vi "Bind SQL Parameters.vi"   [LabVIEW 2023, in "SQLite DB Operator.lvclass"]
uses:
  SQLite DB Operator.lvclass
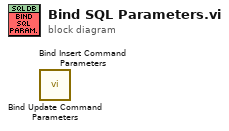
[diagram p0: block diagram]
diagram:
  n1 = call "Bind Update Command Parameters.vi"() -> ()  [unwired: 10 in, 2 out]
  n2 = call "Bind Insert Command Parameters.vi"() -> ()  [unwired: 10 in, 2 out]
